vi "Get All DIDPID Properties.vi"(8 "error in (no error)":errorcluster, 10 "PID Inputs GUID":string, 11 "Section Ref out in":T1 format="%.0x") -> (0 "error out":errorcluster, 2 "DIDPID Array":T2[](array[typedef]) {"Signals"."Byte Order" items=["Little Endian", "Big Endian"]; "Signals"."Data Type" items=["Signed", "Unsigned", "IEEE Float"]}, 3 "Section Ref out":T1 format="%.0x")   [LabVIEW 2013, in "Diagnostics Addon Shared.lvlib"]
uses:
  Diagnostics Addon Shared.lvlib
  <vilib>/NI Veristand/Custom Device API/Custom Device Item Ref.ctl
  DIDPID Parameters.ctl
  DIDPID Signal Parameters.ctl
  DIDPID ID FG.vi
  Get Signals from DIDPID.vi
  Signal Parameters FG.vi
  <vilib>/NI Veristand/Custom Device Tools/Custom Device Utility Library/NI VeriStand - Search for Item by GUID.vi
  <vilib>/NI Veristand/Custom Device API/NI VeriStand - Get Item Data.vi
  GUID Lookup.vi
  <vilib>/NI Veristand/Custom Device API/NI VeriStand - Get Item Property.vi
  <vilib>/NI Veristand/Custom Device API/Get Item Property (Variant).vi
  <vilib>/NI Veristand/Custom Device API/NI VeriStand - Get Custom Device Channel Data.vi
  <vilib>/NI Veristand/Custom Device API/NI VeriStand - Get Item Description.vi
  <vilib>/NI Veristand/Custom Device Tools/Custom Device Utility Library/Custom Device Utility Library.lvlib
  <vilib>/NI Veristand/Custom Device API/Custom Device API.lvlib
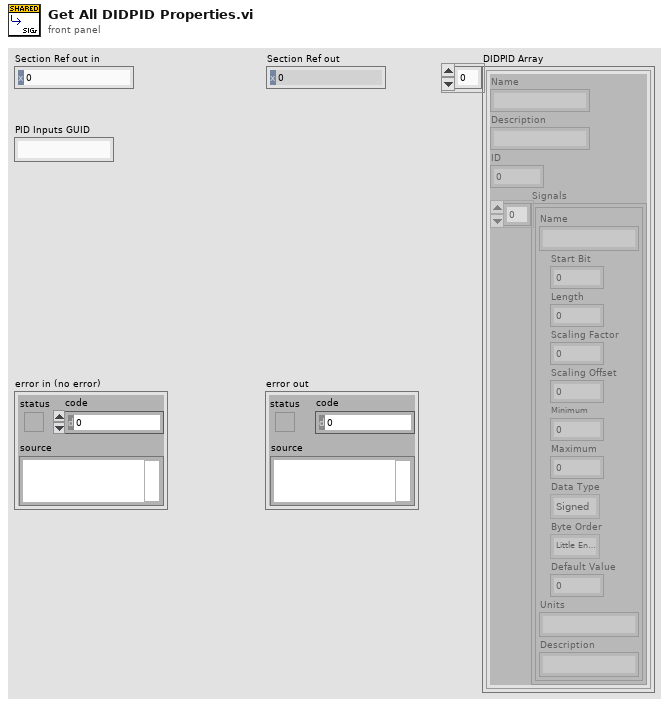
[diagram p1: front panel]
types:
  T1 = typedef "Custom Device API.lvlib/Custom Device Item Ref.ctl" = u64
  T2 = typedef "Diagnostics Addon Shared.lvlib/DIDPID Parameters.ctl" = cluster{"Name":string, "Description":string, "ID":u16, "Signals":T3[]}
  T3 = typedef "Diagnostics Addon Shared.lvlib/DIDPID Signal Parameters.ctl" = cluster{"Name":string, "Start Bit":u8, "Length":u8, "Scaling Factor":dbl, "Scaling Offset":dbl, "Minimum":dbl, "Maximum":dbl, "Data Type":u32, "Byte Order":u32, "Default Value":dbl, "Units":string, "Description":string}
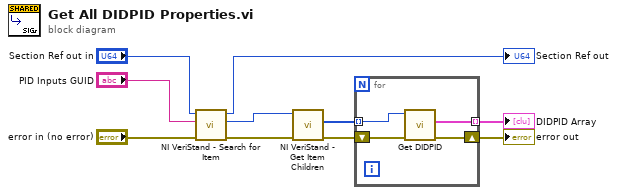
[diagram p0: block diagram]
diagram:
  n1 = call-poly <vilib>:"NI VeriStand - Search for Item.vi"("error in"="error in (no error)", "Item GUID"="PID Inputs GUID", "Section Ref in"="Section Ref out in") -> ("error out"=w4:errorcluster, "Item Ref"=w6:T1, "Section Ref out"=→"Section Ref out":T1)  [unwired: 5 in, 1 out]
  n2 = call <vilib>:"NI VeriStand - Get Item Children.vi"("error in (no error)"=w4, "Item Ref in"=w6) -> ("error out"=w5:errorcluster, "Child Refs"=w7:T1[])  [unwired: 6 in, 2 out]
  n3 = for {
    shift-right: [w13] -> w9
    shift-left: w5 -> [w14]
    tunnel: w7 -> [w12] mode=indexing
    tunnel: [w11] -> w8 mode=indexing
    n4 = call "Get DIDPID.vi"("error in (no error)"=w14, "Item Ref in"=w12) -> ("error out"=w13:errorcluster, "PID In"=w11:T2)  [unwired: 7 in, 1 out]
  }
  "error out" <- w9
  "DIDPID Array" <- w8
